vi "SigSyn (G3)-Set Level (1D).vi"(0 "StimChans In":T1[](array[typedef]) {"Filter"."Stages"."IIR Filter"."Forward Coefficients" format="%.4f"; "Filter"."Stages"."IIR Filter"."Reverse Coefficients" format="%.4f"}, 1 "Apply multiplier? (F)":bool, 5 "Waveform in":dbl[](array[numeric]), 11 "error in (no error)":errorcluster) -> (4 "StimChans Out":T1[](array[typedef]) {"Filter"."Stages"."IIR Filter"."Forward Coefficients" format="%.4f"; "Filter"."Stages"."IIR Filter"."Reverse Coefficients" format="%.4f"}, 6 "Waveform out":dbl[](array[numeric]), 8 "Multiplier":dbl, 10 "Ceiling":dbl, 15 "error out":errorcluster)   [LabVIEW 2015]
uses:
  XControls/Filter (G3)/Filter Type.ctl
  XControls/Filter (G3)/Filter (G3).xctl
  Filter VIs/Filter-Bandwidth Units.ctl
  XControls/Filter (G3)/Filter Data.ctl
  XControls/Level (G3)/Level Units (G3).ctl
  XControls/Level (G3)/Level (G3).xctl
  XControls/Level (G3)/Level Data.ctl
  Controls/Burst XCtl/Burst Data.ctl
  Controls/Burst XCtl/Burst Control.xctl
  Waveform VIs/Pulse Train VIs/Pulse Polarity.ctl
  Waveform VIs/Pulse Train VIs/PT-Continuous State.ctl
  Waveform VIs/Pulse Train VIs/Pulse Train Params.ctl
  Waveform VIs/Noise VIs/Noise (G3).Properties.ctl
  Waveform VIs/Noise VIs/Noise (G3).Data.ctl
  Waveform VIs/Noise VIs/Noise (G3).ctl
  Waveform VIs/File VIs/StimFile-Params.ctl
  Waveform VIs/FM Sweep VIs/FM Sweep Params.ctl
  Waveform VIs/Chirp Train VIs/Chirp Train Params.ctl
  Waveform VIs/Chirp Train VIs/Chirp Train.ctl
  Waveform VIs/Complex Tone VIs/CT-Phase Enum.ctl
  Waveform VIs/Complex Tone VIs/CT-Params.ctl
  Waveform VIs/Complex Tone VIs/CT-Runtime Data.ctl
  XControls/Waveform XControls/Waveform (G3)/Waveform Data.ctl
  XControls/Waveform XControls/Waveform (G3)/Waveform (G3).xctl
  XControls/Advanced Options (G3)/Advanced Options (G3).ctl
  XControls/Advanced Options (G3)/Advanced Options (G3).xctl
  Modulation VIs/SAM VIs/SAM Params.ctl
  Typedefs/Destination.ctl
  XControls/Stimulus Channel (G3)/Full Stimulus Channel Data.ctl
  XControls/Stimulus Channel (G3)/Stimulus Channel (G3).xctl
  XControls/Waveform XControls/Tone (G3)/Tone.Properties.ctl
  XControls/Waveform XControls/Tone (G3)/Tone (G3).xctl
  Waveform VIs/Waveform Enum (V3).ctl
  XControls/Waveform XControls/FM Tone/Data.ctl
  XControls/Waveform XControls/FM Tone/FM Tone.xctl
  XControls/Waveform XControls/Vowel/Vowel.Properties.ctl
  XControls/Waveform XControls/Vowel/Vowel.xctl
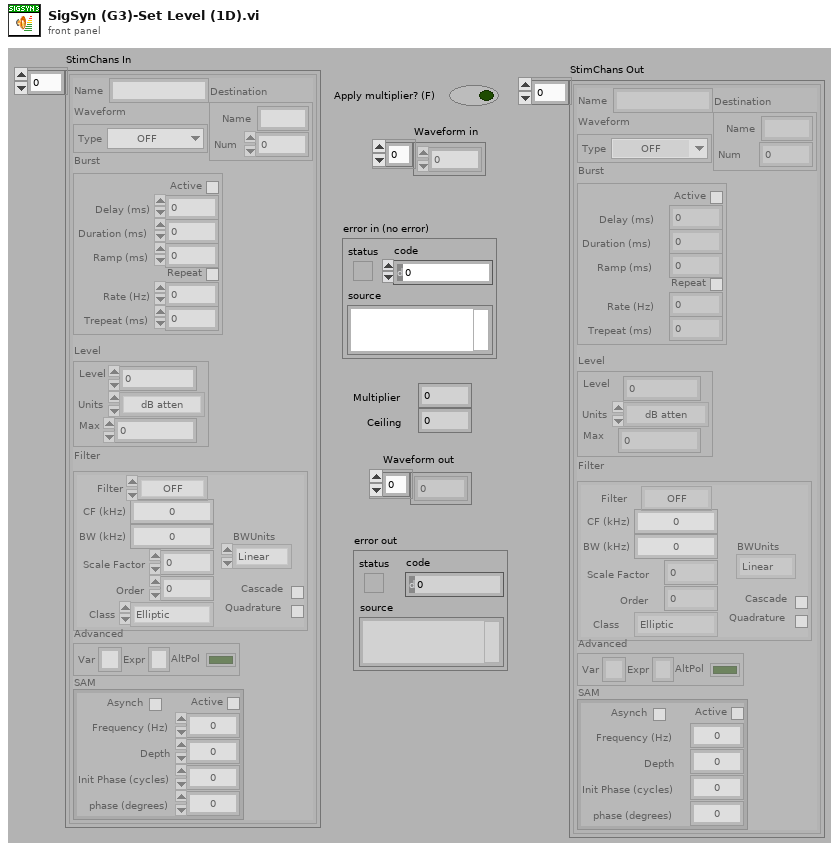
[diagram p1: front panel]
types:
  T1 = typedef "Stimulus Channel (G3).xctl/Full Stimulus Channel Data.ctl" = cluster{"Waveform":T2, "Filter":T20, "Burst":T23, "Level":T24, "Name":string, "Advanced":T26, "SAM":T27, "Destination":T28}
  T2 = typedef "Waveform (G3).xctl/Waveform Data.ctl" = cluster{"Type":T3, "Tone":T4, "Pulse Train":T5, "Noise":T8, "File":T11, "FMSweep":T12, "Chirp Train":T13, "Complex Tone":cluster{"Params":T15, "Data":T17}, "FM":T18, "Vowel":T19}
  T3 = typedef "Waveform Enum (V3).ctl" = enum16{"OFF", "Tone", "Noise", "Pulse Train", "File", "FM Sweep", "Chirp Train", "Complex Tone", "FM Tone", "Vowel"}
  T4 = typedef "Tone (G3).xctl/Tone.Properties.ctl" = cluster{"Frequency (kHz)":dbl, "Phase (cycles)":dbl, "Random phase":bool}
  T5 = typedef "Pulse Train Params.ctl" = cluster{"Pulse width (us)":dbl, "Pulse rate (Hz)":dbl, "Gap (ms)":dbl, "Polarity":T6, "PT State":T7, "Asynch":bool}
  T6 = typedef "Pulse Polarity.ctl" = enum16{"POS", "NEG", "POS-NEG", "NEG-POS"}
  T7 = typedef "PT-Continuous State.ctl" = cluster{"Template":dbl[], "Nperiod":i32, "Index":i32, "Pulse Rate (Hz)":dbl, "Phase (cycles)":dbl, "Noff":i32}
  T8 = typedef "Noise (G3).ctl" = cluster{"Properties":T9, "Data":T10}
  T9 = typedef "Noise (G3).Properties.ctl" = cluster{"InvFilt":bool, "Aweight":bool, "Seed":i32, "Tokens":i32}
  T10 = typedef "Noise (G3).Data.ctl" = cluster{"TokenNum":i32}
  T11 = typedef "StimFile-Params.ctl" = cluster{"Filename":path, "Signal":dbl[], "Channel":i32}
  T12 = typedef "FM Sweep Params.ctl" = cluster{"Rate (oct/s)":dbl, "Fmin (Hz)":dbl, "Fmax (Hz)":dbl, "Ramp (ms)":dbl, "Linear":bool}
  T13 = typedef "Chirp Train.ctl" = cluster{"Params":T14, "Data":cluster{"WF":dbl[]}}
  T14 = typedef "Chirp Train Params.ctl" = cluster{"Fmin (kHz)":dbl, "Fmax (kHz)":dbl, "Compensate":bool, "Duration (ms)":dbl}
  T15 = typedef "CT-Params.ctl" = cluster{"F0 (Hz)":dbl, "Band":cluster{"Flow (Hz)":dbl, "Fhigh (Hz)":dbl}, "Phase":T16, "Min F0 (Hz)":dbl, "Max F0 (Hz)":dbl, "ContinRandPhase":bool, "Max peak factor":dbl, "Max mod depth":dbl, "MinHarmNum":i32, "MaxHarmNum":i32, "Level Mode":enum16{"per component", "overall rms"}}
  T16 = typedef "CT-Phase Enum.ctl" = enum16{"Cosine", "Random", "Alternating"}
  T17 = typedef "CT-Runtime Data.ctl" = cluster{"Ncomp":i32, "MinHarm":i32, "Phase":dbl[], "Amplitude":dbl[], "Npts/frame":i32, "Last F0":dbl, "Fmin":dbl, "Fmax":dbl, "Lslope":dbl, "randphase":bool, "overall rms":bool}
  T18 = typedef "FM Tone.xctl/Data.ctl" = cluster{"Carrier (kHz)":dbl, "ModRate (Hz)":dbl, "Depth (Hz)":dbl, "Phase (cycles)":dbl}
  T19 = typedef "Vowel.xctl/Vowel.Properties.ctl" = cluster{"Freqs":string, "Set level":enum16{"Total", "Per component"}, "Freq":dbl[], "weights":dbl[]}
  T20 = typedef "Filter (G3).xctl/Filter Data.ctl" = cluster{"Type":T21, "CF (kHz)":dbl, "BW (kHz)":dbl, "Cascade":bool, "Quadrature":bool, "Scale Factor":dbl, "Stages":cluster{"IIR Filter":cluster{"filter structure":enum32{"IIR 2nd Order", "IIR 4th Order"}, "Reverse Coefficients":dbl[], "Forward Coefficients":dbl[]}, "State":dbl[]}[], "Class":enum16{"Elliptic", "Butterworth"}, "Order":i32, "BWUnits":T22}
  T21 = typedef "Filter (G3).xctl/Filter Type.ctl" = enum16{"OFF", "Lowpass", "Highpass", "Bandpass", "Bandstop"}
  T22 = typedef "Filter-Bandwidth Units.ctl" = enum16{"Linear", "Octaves"}
  T23 = typedef "Burst Control.xctl/Burst Data.ctl" = cluster{"Active":bool, "Delay (ms)":dbl, "Duration (ms)":dbl, "Ramp (ms)":dbl, "Rate (Hz)":dbl, "Trepeat (ms)":dbl, "Repeat":bool}
  T24 = typedef "Level (G3).xctl/Level Data.ctl" = cluster{"Level":dbl, "Units":T25, "Max":dbl, "Data":cluster{"Multiplier":dbl, "Cal File":path, "Cal":cluster{"Freq (Hz)":dbl[], "Mag (dB SPL)":dbl[], "Phase (deg)":dbl[]}, "audiogram":path}}
  T25 = typedef "Level (G3).xctl/Level Units (G3).ctl" = enum16{"dB atten", "dB SPL", "dB re 1 Vrms", "dB V/Hz½", "dB SL", "mW", "Volts"}
  T26 = typedef "Advanced Options (G3).xctl/Advanced Options (G3).ctl" = cluster{"AltPol":bool, "Var":string, "Expr":string}
  T27 = typedef "SAM Params.ctl" = cluster{"Active":bool, "Frequency (Hz)":dbl, "Depth":dbl, "Init Phase (cycles)":dbl, "phase (degrees)":dbl, "Asynch":bool}
  T28 = typedef "Destination.ctl" = cluster{"Name":string, "Num":i32}
  T29 = typedef "Level XCtl.xctl/Level Data.ctl" = cluster{"Level":dbl, "Units":T30, "Max":dbl, "Multiplier":dbl, "Cal File":path, "Cal":cluster{"Freq (Hz)":dbl[], "Mag (dB SPL)":dbl[], "Phase (deg)":dbl[]}}
  T30 = typedef "Level Units.ctl" = enum16{"dB atten", "dB SPL", "dB re 1 Vrms", "dB V/Hz½", "mW", "dB SL"}
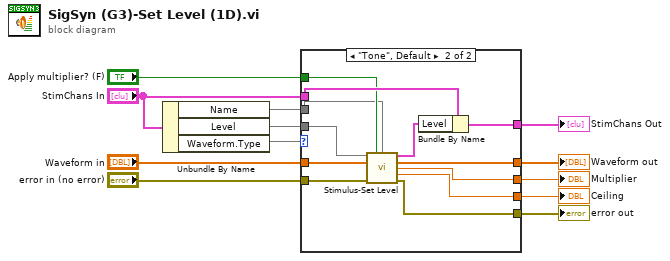
[diagram p0: block diagram]
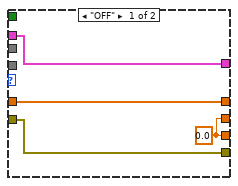
[diagram p2: hidden frame]
diagram:
  n1 = Unbundle By Name("StimChans In") -> ("Name"=w2, "Level"=w10, "Waveform.Type"=w1)
  n2 = case shown="\"Tone\", Default" w1 {
    tunnel: "Waveform in" -> [w14 w28]
    tunnel: "error in (no error)" -> [w15 w27]
    tunnel: w10 -> [_ w26]
    tunnel: [w16 w25] -> w9
    tunnel: "StimChans In" -> [w16 w24]
    tunnel: [w14 w22] -> w7
    tunnel: "Apply multiplier? (F)" -> [_ w21]
    tunnel: [w13 w20] -> w5
    tunnel: [w13 w19] -> w4
    tunnel: [w15 w18] -> w3
    tunnel: w2 -> [_ w17]
    frame "OFF" {
      w13 = 0.0 ("Ceiling")
    }
    frame "Tone", Default {
      n3 = call "Stimulus-Set Level.vi"("Level"=w26, "Apply multiplier? (F)"=w21, "Name"=w17, "Waveform in"=w28, "error in (no error)"=w27) -> ("Level out"=w23:T29, "Waveform out"=w22:dbl[], "Multiplier"=w20:dbl, "Ceiling"=w19:dbl, "error out"=w18:errorcluster)  [unwired: 6 in]
      n4 = Bundle By Name(cluster=w24, "Level"=w23) -> (w25:cluster{})
    }
  }
  "error out" <- w3
  "StimChans Out" <- w9
  "Waveform out" <- w7
  "Multiplier" <- w5
  "Ceiling" <- w4
